vi "TransferFunction.vi"() -> ()   [LabVIEW 2018]
uses:
  <vilib>/addons/Control Design/_Model Construction/Model Creation.llb/Model Creation SubVI/cd_Create Transfer Function Model.vi
  <vilib>/addons/Control Design/_Time Response Analysis/Time Response.llb/Time Response subVI/cd_Step Response (Transfer Function).vi
  <vilib>/addons/Control Design/_Utility/Model Viewer.llb/Model Viewer SubVI/cd_Draw Transfer Function Equation (TF).vi
  <vilib>/Analysis/NI_AALPro.lvlib
  <vilib>/addons/Control Design/_Model Construction/NI_LinSys_Model Creation.lvlib
  <vilib>/addons/Control Design/_Utility/NI_CD_Model Viewer.lvlib
  <vilib>/addons/Control Design/_Time Response Analysis/NI_CD_Time Response.lvlib
panel:
  out "Transfer\nFunction\nDisplay":picture
  in  "Sampling\nTime":dbl
  in  "Blower Opening Control at Plant":dbl(slide) scale=0.0..10.0
  out "Polynomial Fit (Fixed)\nfor Temp-Voltage":i32=2
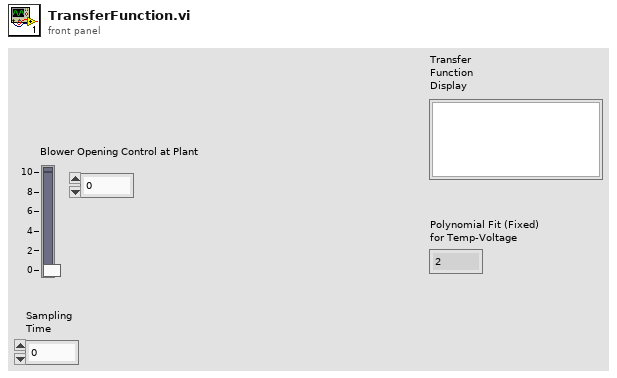
[diagram p1: front panel]
types:
  T1 = typedef "NI_LinSys_Model Typedefs.lvlib/CD Transfer Function Model (MIMO).ctl" = cluster{"properties":T2, "transfer function(s)":T3[][]}
  T2 = typedef "NI_LinSys_Model Typedefs.lvlib/CD General Elements.ctl" = cluster{"Model name":string, "Input names":string[], "Output names":string[], "Input Delays":dbl[], "Output Delays":dbl[], "Sampling Time":dbl, "Notes":string}
  T3 = typedef "NI_LinSys_Model Typedefs.lvlib/CD Transfer Function Model (SISO).ctl" = cluster{"Numerator":dbl[], "Denominator":dbl[], "delay":dbl}
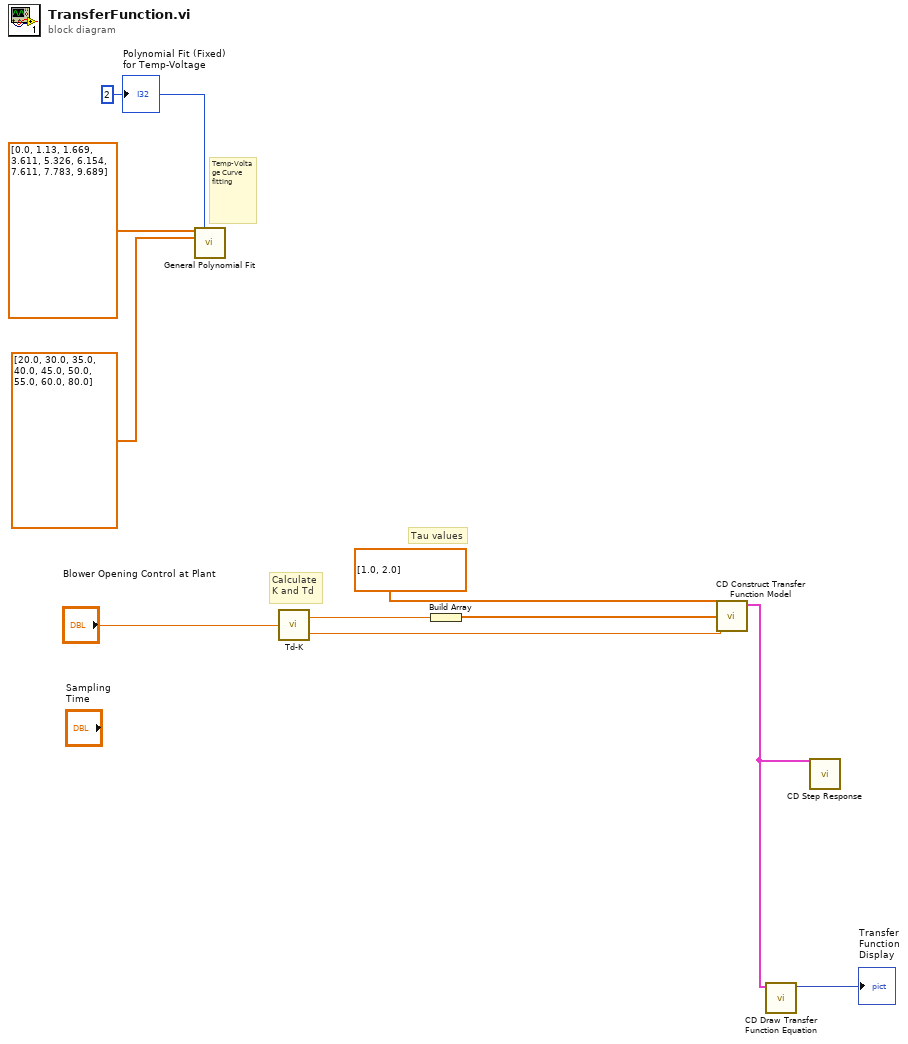
[diagram p0: block diagram]
diagram:
  w8 = 2
  # "Tau values"
  # "Calculate\nK and Td"
  # "Temp-Voltage Curve fitting"
  n1 = call <vilib>:"General Polynomial Fit.vi"("Y"=dbl[] [0.0, 1.13, 1.669, 3.611, 5.326, 6.154, 7.611, 7.783, 9.689], "polynomial order"=w8, "X"=dbl[] [20.0, 30.0, 35.0, 40.0, 45.0, 50.0, 55.0, 60.0, 80.0]) -> ()  [unwired: 9 in, 4 out]
  n2 = call "Td-K.vi"("Blower Opening \nInput (Degrees)"="Blower Opening Control at Plant") -> ("K Calculated"=w5:dbl, "Tau-d Calculated"=w6:dbl)
  n3 = Build Array(w5) -> (w4:dbl[])
  n4 = call-poly <vilib>:"CD Construct Transfer Function Model.vi"("Delay"=w6, "Denominator"=dbl[] [1.0, 2.0], "Numerator"=w4) -> ("Transfer Function Model"=w1:T1)  [unwired: 7 in, 1 out]
  n5 = call-poly <vilib>:"CD Draw Transfer Function Equation.vi"("Transfer Function Model"=w1) -> ("Equation"=→"Transfer\nFunction\nDisplay":picture)  [unwired: 8 in, 2 out]
  n6 = call-poly <vilib>:"CD Step Response.vi"("Transfer Function Model"=w1) -> ()  [unwired: 8 in, 3 out]
  "Polynomial Fit (Fixed)\nfor Temp-Voltage" <- w8
